vi "configure.vi"(0 "identifier":string, 1 "Board":u16, 2 "fast_filter_thr":u32, 3 "energy_filter_thr":u32, 4 "energy_baseline_thr":u32, 5 "max_risetime":dbl, 6 "gain":dbl, 7 "error in (no error)":errorcluster, 8 "peaking_time":u32, 9 "max_peaking_time":u32, 10 "flat_top":u32, 11 "edge_peaking_time":u32, 12 "edge_flat_top":u32, 13 "reset_recovery_time":u32, 14 "zero_peak_freq":dbl, 15 "baseline_samples":u32, 16 "inverted_input":bool, 17 "time_constant":dbl, 18 "base_offset":u32, 19 "overflow_recovery":u32, 24 "other_param":u32, 25 "tail_coefficient":dbl, 26 "reset_threshold":u32) -> (20 "function return":u32, 27 "error out":errorcluster)   [LabVIEW 2015, in "XGL_DPP.lvlib"]
doc: "EXTERN DECLSPEC uint32_t CALL_CONV configure(const char * identifier, uint16_t Board, const configuration cfg);"
uses:
  XGL_DPP.lvlib
  XGL_DPP.dll
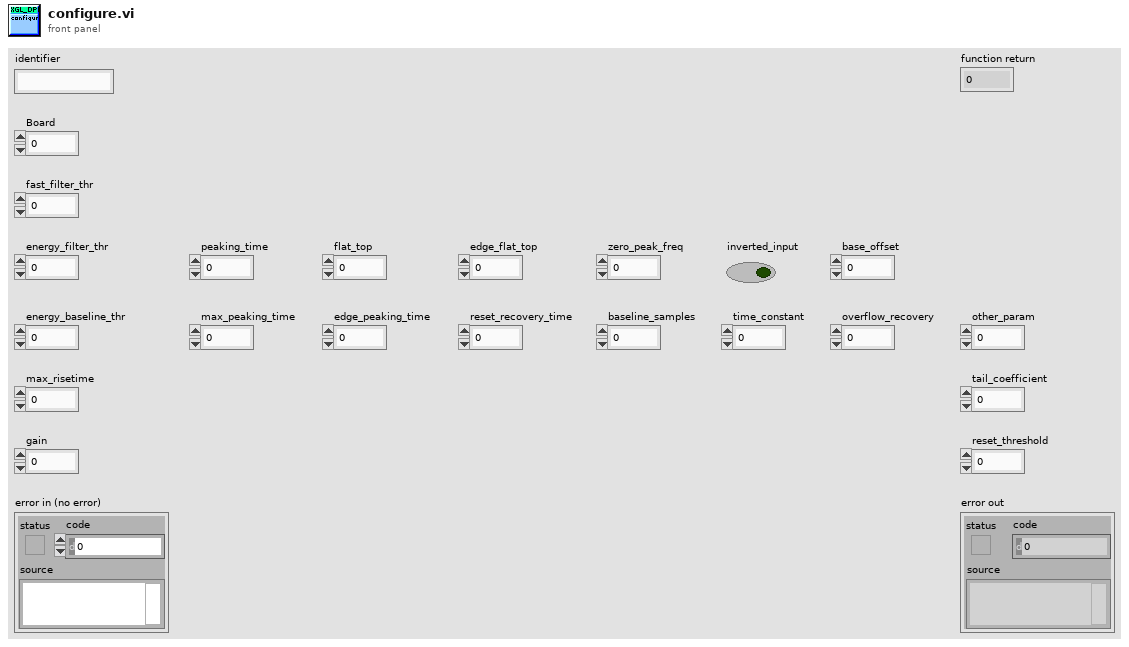
[diagram p1: front panel]
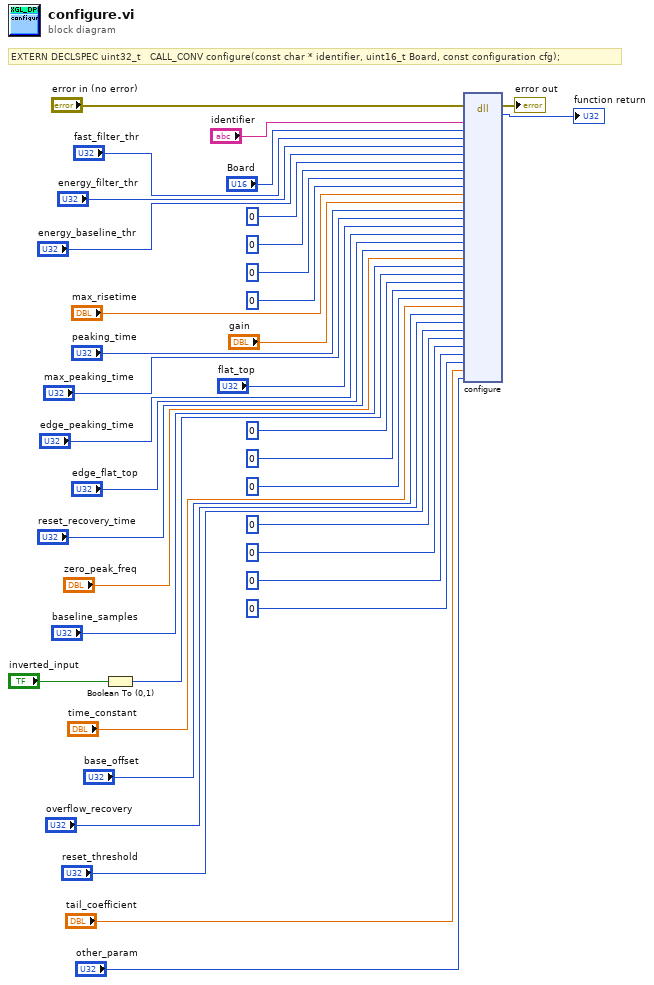
[diagram p0: block diagram]
diagram:
  # "EXTERN DECLSPEC uint32_t   CALL_CONV configure(const char * identifier, uint16_t Board, const configuration cfg);"
  n1 = Boolean To (0,1)(Boolean="inverted_input") -> (0, 1=w16:i16)
  n2 = dll-call lib="D:/Users/XRF/Desktop/Scanning Software_Demokritos_2015_v7/libs/Vis_2/XGL_DPP.*" fn="configure"(error in="error in (no error)", "identifier"="identifier", "Board"="Board", "fast_filter_thr"="fast_filter_thr", "energy_filter_thr"="energy_filter_thr", "energy_baseline_thr"="energy_baseline_thr", "@dummy control@"=i8 0, "@dummy control@"=i8 0, "@dummy control@"=i8 0, "@dummy control@"=i8 0, "max_risetime"="max_risetime", "gain"="gain", "peaking_time"="peaking_time", "max_peaking_time"="max_peaking_time", "flat_top"="flat_top", "edge_peaking_time"="edge_peaking_time", "edge_flat_top"="edge_flat_top", "reset_recovery_time"="reset_recovery_time", "zero_peak_freq"="zero_peak_freq", "baseline_samples"="baseline_samples", "inverted_input"=w16, "@dummy control@"=i8 0, "@dummy control@"=i8 0, "@dummy control@"=i8 0, "time_constant"="time_constant", "base_offset"="base_offset", "overflow_recovery"="overflow_recovery", "reset_threshold"="reset_threshold", "@dummy control@"=i8 0, "@dummy control@"=i8 0, "@dummy control@"=i8 0, "@dummy control@"=i8 0, "tail_coefficient"="tail_coefficient", "other_param"="other_param") -> (error out=→"error out":errorcluster, →"function return":u32)  [unwired: 35 in, 1 out]
